vi "Configure Measurement Core.vi"(7 "range (-1.0: Auto)":dbl=-1.0 format="%^.2e", 8 "error in (no error)":errorcluster, 9 "absolute resolution (0.001)":dbl=0.001 format="%^.2e", 10 "measurement function (DC Volts)":i32(ring)=1 items=["DC Volts"=1, "AC Volts"=2, "DC Current"=3, "AC Current"=4, "2 Wire Resistance"=5, "4 Wire Resistance"=101, "AC + DC Volts"=106, "AC + DC Current"=107, "Frequency"=104, "Period"=105, "Temperature"=108], 11 "IVI_DMM in":refnum<class "IVI_DMM.lvclass">) -> (0 "error out":errorcluster, 3 "IVI_DMM out":refnum<class "IVI_DMM.lvclass">)   [LabVIEW 2016, in "IVI_DMM.lvlib" / "IVI_DMM.lvclass"]
doc: "This VI configures the common properties of the DMM. These properties include the measurement function, maximum range, and resolution."
uses:
  IVI_DMM.lvclass
  IVI_DMM.lvclass/IVI_DMM.ctl
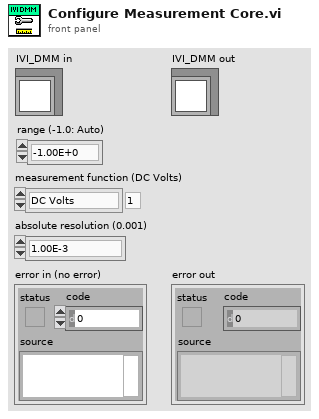
[diagram p1: front panel]
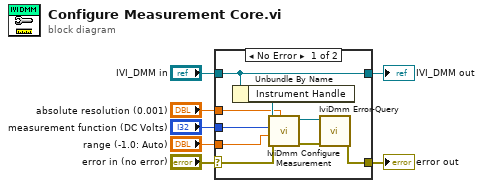
[diagram p0: block diagram]
diagram:
  n1 = case shown="No Error" "error in (no error)" {
    selector: "error in (no error)" -> [w11 w18]
    tunnel: [w9 w18] -> w6
    tunnel: [w16 w17] -> w4
    tunnel: "IVI_DMM in" -> [w16 w17]
    tunnel: "absolute resolution (0.001)" -> [w14 _]
    tunnel: "measurement function (DC Volts)" -> [w13 _]
    tunnel: "range (-1.0: Auto)" -> [w12 _]
    frame No Error {
      n2 = Unbundle By Name(w16) -> ("Instrument Handle"=w15:refnum<k15>)
      n3 = call <vilib>:"IviDmm Configure Measurement.vi"("absolute resolution (0.001)"=w14, "error in (no error)"=w11, "range (-1.0: Auto)"=w12, "measurement function (DC Volts)"=w13, "instrument handle"=w15) -> ("error out"=w10:errorcluster, "instrument handle out"=w8:refnum<k15>)  [unwired: 5 in]
      n4 = call <vilib>:"IviDmm Error-Query.vi"("error in (no error)"=w10, "instrument handle"=w8) -> ("error out"=w9:errorcluster)  [unwired: 6 in, 3 out]
    }
    frame Error {
    }
  }
  "error out" <- w6
  "IVI_DMM out" <- w4
